vi "Synchronization Trigger Constants.vi"() -> (4 "Sync Pulse":string(combo)="PXI_Trig0", 6 "Start Trigger":string(combo)="PXI_Trig0", 8 "Start Trigger Edge":i32(ring)=10280 items=["Rising"=10280, "Falling"=10171])   [LabVIEW 2020]
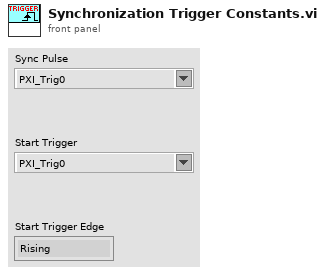
[diagram p1: front panel]
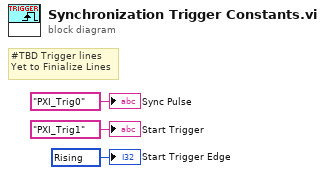
[diagram p0: block diagram]
diagram:
  w1 = 10280 items=["Rising"=10280, "Falling"=10171] ("Start Trigger Edge")
  # "#TBD Trigger lines\nYet to Finialize Lines"
  "Sync Pulse" <- "PXI_Trig0" ("Sync Pulse")
  "Start Trigger" <- "PXI_Trig1" ("Start Trigger")
  "Start Trigger Edge" <- w1
